vi "(MATRICE)_Converto virgolo_punti e punti_virgole.vi"(1 "Stringa Input":string) -> (0 "appended array":dbl[](array[numeric]))   [LabVIEW 2012]
panel:
  out "result string":string
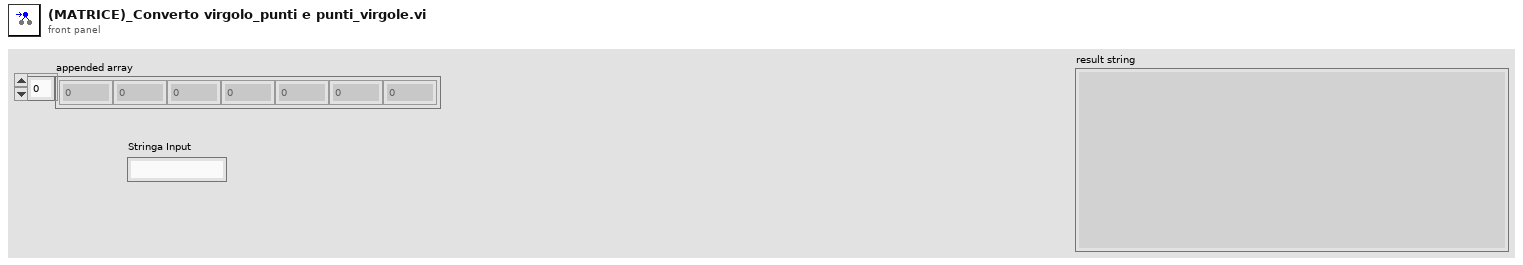
[diagram p1: front panel]
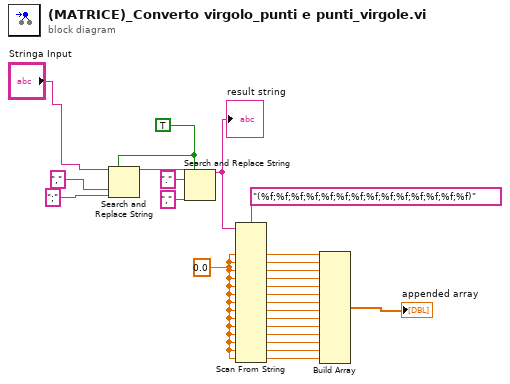
[diagram p0: block diagram]
diagram:
  w17 = TRUE
  w20 = 0.0
  n1 = Search and Replace String(replace all?=w17, input string="Stringa Input", search string=",", replace string=";" ("replace string (\"\")")) -> (result string=w23:string)  [unwired: 4 in, 3 out]
  n2 = Search and Replace String(replace all?=w17, input string=w23, search string=".", replace string="," ("replace string (\"\")")) -> (result string=w19:string)  [unwired: 4 in, 3 out]
  "result string" <- w19
  n3 = Scan From String(format string="(%f;%f;%f;%f;%f;%f;%f;%f;%f;%f;%f;%f;%f;%f)", input string=w19, default 1=w20, default 2=w20, default 3=w20, default 4=w20, default 5=w20, default 6=w20, default 7=w20, default 8=w20, default 9=w20, default 10=w20, default 11=w20, default 12=w20, default 13=w20, default 14=w20) -> (output 1=w15:dbl, output 2=w14:dbl, output 3=w13:dbl, output 4=w12:dbl, output 5=w11:dbl, output 6=w10:dbl, output 7=w9:dbl, output 8=w8:dbl, output 9=w7:dbl, output 10=w6:dbl, output 11=w5:dbl, output 12=w4:dbl, output 13=w3:dbl, output 14=w2:dbl)  [unwired: 2 in, 3 out]
  n4 = Build Array(w15, w14, w13, w12, w11, w10, w9, w8, w7, w6, w5, w4, w3, w2) -> (→"appended array":dbl[])
